vi "Set Window Color to Transparent.vi"(4 "Calling VI's reference":refnum<vi>, 5 "error in (no error)":errorcluster, 6 "Activate":bool=TRUE, 7 "Color to Replace":u32(colorbox)=16777238, 8 "Factor":u8=255) -> (0 "error out":errorcluster)   [LabVIEW 2011]
uses:
  user32.dll
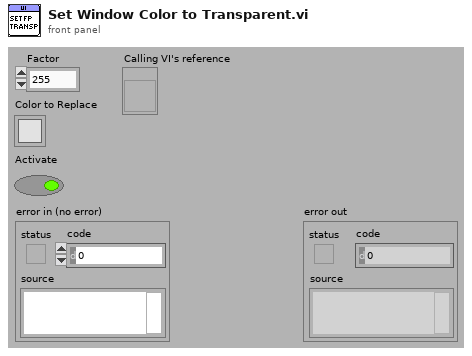
[diagram p1: front panel]
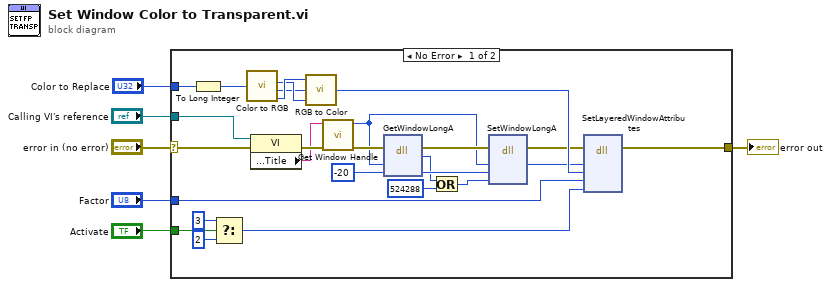
[diagram p0: block diagram]
diagram:
  n1 = case shown="No Error" "error in (no error)" {
    selector: "error in (no error)" -> [w8 w33]
    tunnel: "Activate" -> [w22 _]
    tunnel: "Calling VI's reference" -> [w19 _]
    tunnel: "Factor" -> [w12 _]
    tunnel: "Color to Replace" -> [w11 _]
    tunnel: [w9 w33] -> w2
    frame No Error {
      n2 = To Long Integer(number=w11) -> (32bit integer=w29:i32)
      n3 = Select(t=3, s=w22, f=2) -> (s? t:f=w23:i32)
      n4 = call <vilib>:"Color to RGB.vi"("Color"=w29) -> ("R"=w27:u8, "G"=w26:u8, "B"=w28:u8)  [unwired: 1 out]
      n5 = property class="VI"(reference=w19, error in=w8) -> (error out=w20:errorcluster, "Front Panel.Title"=w18:string)  [unwired: 1 out]
      n6 = call <vilib>:"RGB to Color.vi"("B"=w27, "G"=w26, "R"=w28) -> ("Color"=w30:u32)
      n7 = call "Get Window Handle.vi"("error in"=w20, "Window Name In"=w18) -> ("error out"=w21:errorcluster, "Window Handle Out"=w7:u32)  [unwired: 1 in, 3 out]
      n8 = dll-call lib="user32.dll" fn="GetWindowLongA" label="getWindowLong"(error in=w21, "handle"=w7, "nIndex"=-20) -> (error out=w14:errorcluster, w16:i32, "nIndex"=w32:i32)  [unwired: 3 in, 1 out]
      n9 = Or(x=w16, y=524288) -> (x .or. y?=w13:i32)
      n10 = dll-call lib="user32.dll" fn="SetWindowLongA" label="SetWindowLong"(error in=w14, "handle"=w7, "nIndex"=w32, "dwNewLong"=w13) -> (error out=w15:errorcluster, "handle"=w10:i32)  [unwired: 4 in, 2 out]
      n11 = dll-call lib="user32.dll" fn="SetLayeredWindowAttributes" label="SetLayerdWindowAttributs"(error in=w15, "handle"=w10, "crkey"=w30, "bAlpha"=w12, "dwFlags"=w23) -> (error out=w9:errorcluster)  [unwired: 5 in, 3 out]
    }
    frame Error {
    }
  }
  "error out" <- w2
